vi "AO Clear.vi"(0 "error in (no error)":errorcluster, 4 "taskID in":u32 format="%x") -> (3 "error out":errorcluster, 7 "taskID out":u32 format="%x")   [LabVIEW 2009]
doc: "Clears the analog output task associated with <B>taskID in</B>."
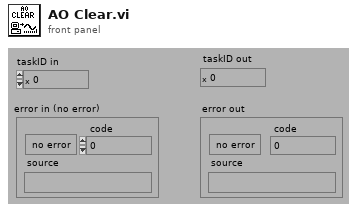
[diagram p1: front panel]
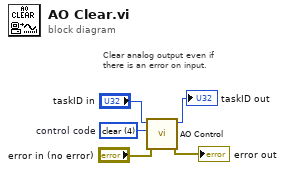
[diagram p0: block diagram]
diagram:
  w1 = u16 4 items=["start", "pause", "pause at EOC", "resume", "clear", "switch to next buffer", "switch to next buffer at EOC", "new staging list"]  # control code
  # "Clear analog output even if there is an error on input."
  n1 = call "AO Control.vi"("error in (no error)"="error in (no error)", "control code (0: start)"=w1, "task ID"="taskID in") -> ("error out"=→"error out":errorcluster, "task ID out"=→"taskID out":u32)  [unwired: 7 in]
